vi "LED Lights Global.vi"() -> ()   [LabVIEW 2015]
uses:
  NavX Light Global Type Def.ctl
  Drive Global Type Def.ctl
  Master Slave Drive Motors Type Def.ctl
  Motor Global Type Def.ctl
panel:
  out "LED Lights Vision":bool
  in  "Drive Subsystem Global":T1
  in  "NavX Global":T4
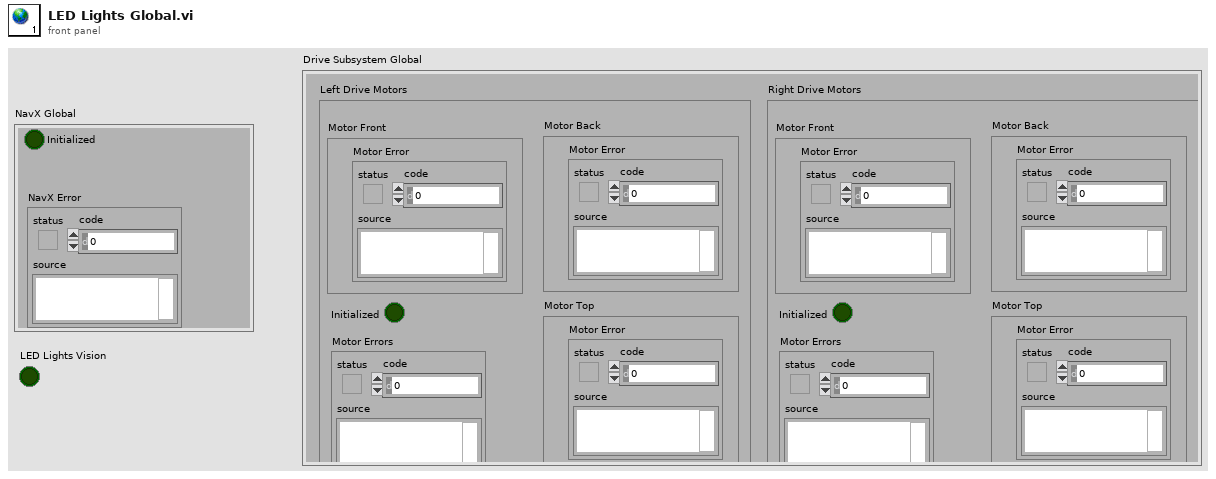
[diagram p1: front panel]
types:
  T1 = typedef "Drive Global Type Def.ctl" = cluster{"Left Drive Motors":T2, "Right Drive Motors":T2}
  T2 = typedef "Master Slave Drive Motors Type Def.ctl" = cluster{"Motor Front":T3, "Motor Back":T3, "Motor Errors":errorcluster, "Motor Top":T3, "Initialized":bool}
  T3 = typedef "Motor Global Type Def.ctl" = cluster{"Motor Error":errorcluster}
  T4 = typedef "NavX Light Global Type Def.ctl" = cluster{"NavX Error":errorcluster, "Initialized":bool}
diagram:
